vi "Send Inner Event.vi"(8 "error in (no error)":errorcluster, 10 "CEID":u32, 11 "Scenarios Class in":refnum<class "Scenarios Class.lvclass">) -> (0 "error out":errorcluster, 3 "Scenarios Class out":refnum<class "Scenarios Class.lvclass">)   [LabVIEW 2020, in "SECS Scenarios.lvlib" / "Scenarios Class.lvclass"]
uses:
  Scenarios Class.lvclass
  07-Event Report From Equipment/07-Event Report From Equipment.lvclass
  D:/Dropbox/SECS/SECS_GEM v1.1.0/Com/SECS Scenarios/Scenarios Class/Scenarios Class.lvclass
  Scenarios Class.lvclass/Scenarios Class.ctl
  07-Event Report From Equipment/07-Event Report From Equipment.lvclass/07-Event Report From Equipment.ctl
  07-Event Report From Equipment/Write CEID.vi
  Write HSMS Class.vi
  Read Reply State.vi
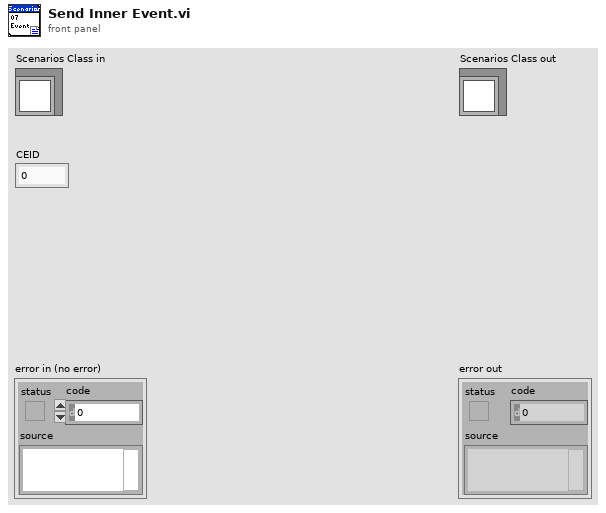
[diagram p1: front panel]
types:
  T1 = typedef "SECS Scenarios.lvlib/Scenarios Class.lvclass/Reply State.ctl" = enum16{"OK", "Illegal Data", "Unknown Stream", "Unknown Function", "Off-Line", "T3 Timeout", "Inner-Timeout"}
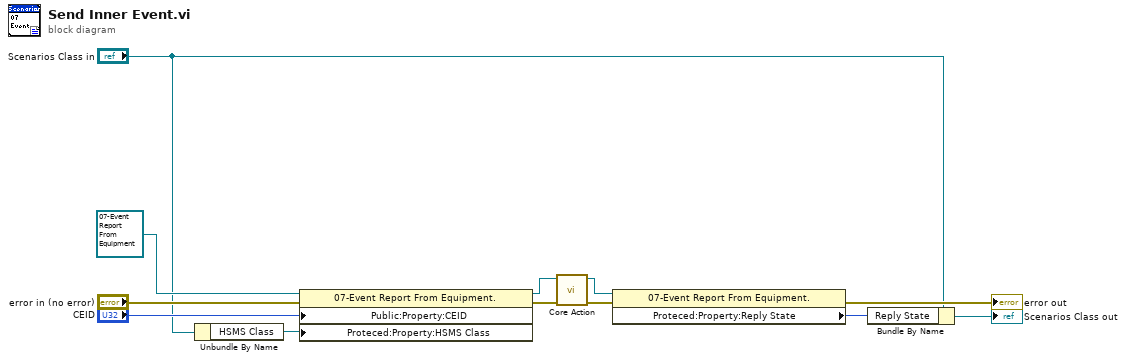
[diagram p0: block diagram]
diagram:
  n1 = Unbundle By Name("Scenarios Class in") -> ("HSMS Class"=w1:refnum<class "HSMS Class.lvclass">)
  n2 = property class="07-Event Report From Equipment."(reference=refnum<class "07-Event Report From Equipment.lvclass"> refnum ("07-Event Report From Equipment in"), error in="error in (no error)", "Public:Property:CEID"="CEID", "Proteced:Property:HSMS Class"=w1) -> (reference out=w8:refnum<class "07-Event Report From Equipment.lvclass">, error out=w9:errorcluster)
  n3 = call-dynamic "Core Action.vi"("error in (no error)"=w9, "07-Event Report From Equipment in"=w8) -> ("error out"=w7:errorcluster, "07-Event Report From Equipment out"=w6:refnum<class "07-Event Report From Equipment.lvclass">)  [unwired: 7 in, 1 out]
  n4 = property class="07-Event Report From Equipment."(reference=w6, error in=w7) -> (error out=→"error out":errorcluster, "Proteced:Property:Reply State"=w5:T1)  [unwired: 1 out]
  n5 = Bundle By Name(cluster="Scenarios Class in", "Reply State"=w5) -> (→"Scenarios Class out":refnum<class "Scenarios Class.lvclass">)
